vi "GetClass.vi"(0 "TSM Context":T1, 11 "error in":errorcluster) -> (4 "GlobalTestData":refnum<class "GlobalTestData.lvclass">, 15 "error out":errorcluster)   [LabVIEW 2019, in "GlobalTestData.lvclass"]
doc: "This function should be called at the start of test code module. It will construct the GlobalTestData class wire by referencing the approprate instance of the Semiconductor Module Context."
uses:
  GlobalTestData.lvclass
  <vilib>/NI_TestStand_SemiconductorModule/NI_TestStand_Semiconductor_Module.lvlibp/PinMap/General/SemiconductorModuleContext.ctl
  GlobalTestData.lvclass/GlobalTestData.ctl
  Private/PersistantClassData.vi
  <vilib>/NI_TestStand_SemiconductorModule/NI_TestStand_Semiconductor_Module.lvlibp
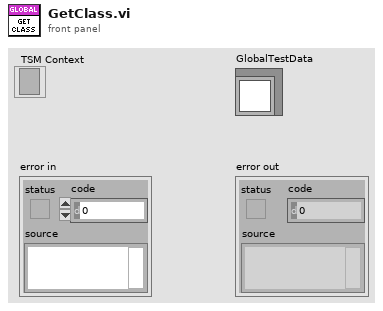
[diagram p1: front panel]
types:
  T1 = typedef "NI_TestStand_Semiconductor_Module.lvlibp/SemiconductorModuleContext.ctl" = refnum<k7>
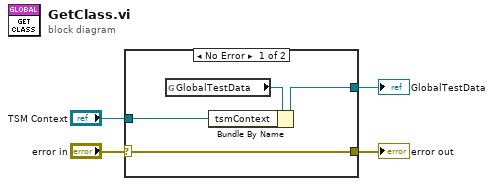
[diagram p0: block diagram]
diagram:
  n1 = case shown="No Error" "error in" {
    selector: "error in" -> [w6 w9]
    tunnel: [w6 w9] -> w3
    tunnel: [w8 _] -> w2
    tunnel: "TSM Context" -> [w5 _]
    frame No Error {
      n2 = global read "PersistantClassData.vi" "GlobalTestData"() -> (w7:refnum<class "GlobalTestData.lvclass">)
      n3 = Bundle By Name(cluster=w7, "tsmContext"=w5) -> (w8:refnum<class "GlobalTestData.lvclass">)
    }
    frame Error {
    }
  }
  "error out" <- w3
  "GlobalTestData" <- w2
